vi "rechtdoor.vi"   [LabVIEW 2019]
uses:
  <vilib>/myRIO/Common/Instrument Driver Framework/Utilities/typedefs/Analog Scaling Constants.ctl
  <vilib>/myRIO/Common/Instrument Driver Framework/Utilities/typedefs/Analog Scaling Constants List.ctl
  <vilib>/myRIO/Common/Instrument Driver Framework/myRIO v1.0/AO/typedefs/AO Channels Enum.ctl
  <vilib>/myRIO/Common/Instrument Driver Framework/myRIO v1.0/AO/typedefs/AO Channels List.ctl
  <vilib>/myRIO/Common/Instrument Driver Framework/Utilities/typedefs/Generic FPGA Reference.ctl
  <vilib>/myRIO/Common/Instrument Driver Framework/Utilities/typedefs/myRIO v1.0 Reference.ctl
  <vilib>/myRIO/Common/Instrument Driver Framework/Utilities/typedefs/Hardware Version Enum.ctl
  <vilib>/myRIO/Common/Instrument Driver Framework/Utilities/typedefs/myRIO Generic Hardware Reference.ctl
  <vilib>/myRIO/Instrument Drivers/Onboard IO/AO/typedefs/AO Reference.ctl
  <vilib>/myRIO/Instrument Drivers/Onboard IO/AO/AO.lvlib
  <vilib>/myRIO/Instrument Drivers/Onboard IO/AO/vis/Write.vi
  <vilib>/userDefined/High Color/nirio_resource_hc.ctl
  <vilib>/myRIO/Common/Instrument Driver Framework/myRIO v1.0/AO/vis/myRIO v1.1 Open AO.vi
  <vilib>/myRIO/Instrument Drivers/Onboard IO/AO/vis/myRIO AO Open.xnode
  <vilib>/myRIO/Common/Instrument Driver Framework/Utilities/vis/Is FPGA Ref Available.vi
  <vilib>/myRIO/Express VI/Onboard IO/AO/AO Express VI.xnode
  <vilib>/myRIO/Common/Instrument Driver Framework/myRIO v1.0/DIO/typedefs/DIO Channels Enum.ctl
  <vilib>/myRIO/Common/Instrument Driver Framework/myRIO v1.0/DIO/typedefs/DIO Channels List.ctl
  <vilib>/myRIO/Instrument Drivers/Onboard IO/DIO/typedefs/DIO Reference.ctl
  <vilib>/myRIO/Instrument Drivers/Onboard IO/DIO/DIO.lvlib
  <vilib>/myRIO/Instrument Drivers/Onboard IO/DIO/vis/Read.vi
  <vilib>/myRIO/Instrument Drivers/Onboard IO/DIO/vis/myRIO DIO Open.xnode
  <vilib>/myRIO/Express VI/Onboard IO/DI/DI Express VI.xnode
  interface.vi
  <vilib>/myRIO/Common/Instrument Driver Framework/myRIO v1.0/DIO/vis/myRIO v1.1 Open DIO.vi
types:
  T1 = typedef "AO.lvlib/AO Reference.ctl" = cluster{"myRIO Reference":T2, "AO Channel List":T6, "AO Scaling Constant List":T8}
  T2 = typedef "myRIO Generic Hardware Reference.ctl" = cluster{"myRIO Model":T3, "myRIO Hardware Reference":T4}
  T3 = typedef "Hardware Version Enum.ctl" = enum16{"Unknown", "myRIO-1900", "myRIO-1950", "roboRIO", "NI ELVIS RIO CM", "ELVIS III"}
  T4 = typedef "myRIO v1.0 Reference.ctl" = cluster{"Generic FPGA Reference":T5, "Allow multiple opens":bool}
  T5 = typedef "Generic FPGA Reference.ctl" = refnum<k20>
  T6 = typedef "AO Channels List.ctl" = T7[]
  T7 = typedef "AO Channels Enum.ctl" = enum16{"Not Connected", "AudioOut/Left", "AudioOut/Right", "C/AO0", "C/AO1", "A/AO0", "A/AO1", "B/AO0", "B/AO1"}
  T8 = typedef "Analog Scaling Constants List.ctl" = T9[]
  T9 = typedef "Analog Scaling Constants.ctl" = cluster{"LSB Weight (Volts)":dbl, "Offset (Volts)":dbl, "Signed?":bool}
  T10 = typedef "nirio_resource_hc.ctl" = tag
  T11 = typedef "DIO.lvlib/DIO Reference.ctl" = cluster{"myRIO Reference":T2, "DIO Channels List":T12}
  T12 = typedef "DIO Channels List.ctl" = T13[]
  T13 = typedef "DIO Channels Enum.ctl" = enum16{"Not Connected", "C/DIO0", "C/DIO1", "C/DIO2", "C/DIO3", "C/DIO4", "C/DIO5", "C/DIO6", "C/DIO7", "A/DIO0", "A/DIO1", "A/DIO2", "A/DIO3", "A/DIO4", "A/DIO5", "A/DIO6", "A/DIO7", "A/DIO8", "A/DIO9", "A/DIO10", "A/DIO11", "A/DIO12", "A/DIO13", "A/DIO14", "A/DIO15", "A/DIO16", "A/DIO17", "A/DIO18", "A/DIO19", "B/DIO0", "B/DIO1", "B/DIO2", "B/DIO3", "B/DIO4", "B/DIO5", "B/DIO6", "B/DIO7", "B/DIO8", "B/DIO9", "B/DIO10", "B/DIO11", "B/DIO12", "B/DIO13", "B/DIO14", "B/DIO15", "B/DIO16", "B/DIO17", "B/DIO18", "B/DIO19", "LED0", "LED1", "LED2", "LED3", "Button0", "DIO/DIO0", "DIO/DIO1", "DIO/DIO2", "DIO/DIO3", "DIO/DIO4", "DIO/DIO5", "DIO/DIO6", "DIO/DIO7", "DIO/DIO8", "DIO/DIO9", "SPI/CS0", "SPI/CS1", "SPI/CS2", "SPI/CS3", "LED RADIO (Green)", "LED RADIO (Red)", "LED COMM (Green)", "LED COMM (Red)", "LED MODE (Green)", "LED MODE (Red)"}
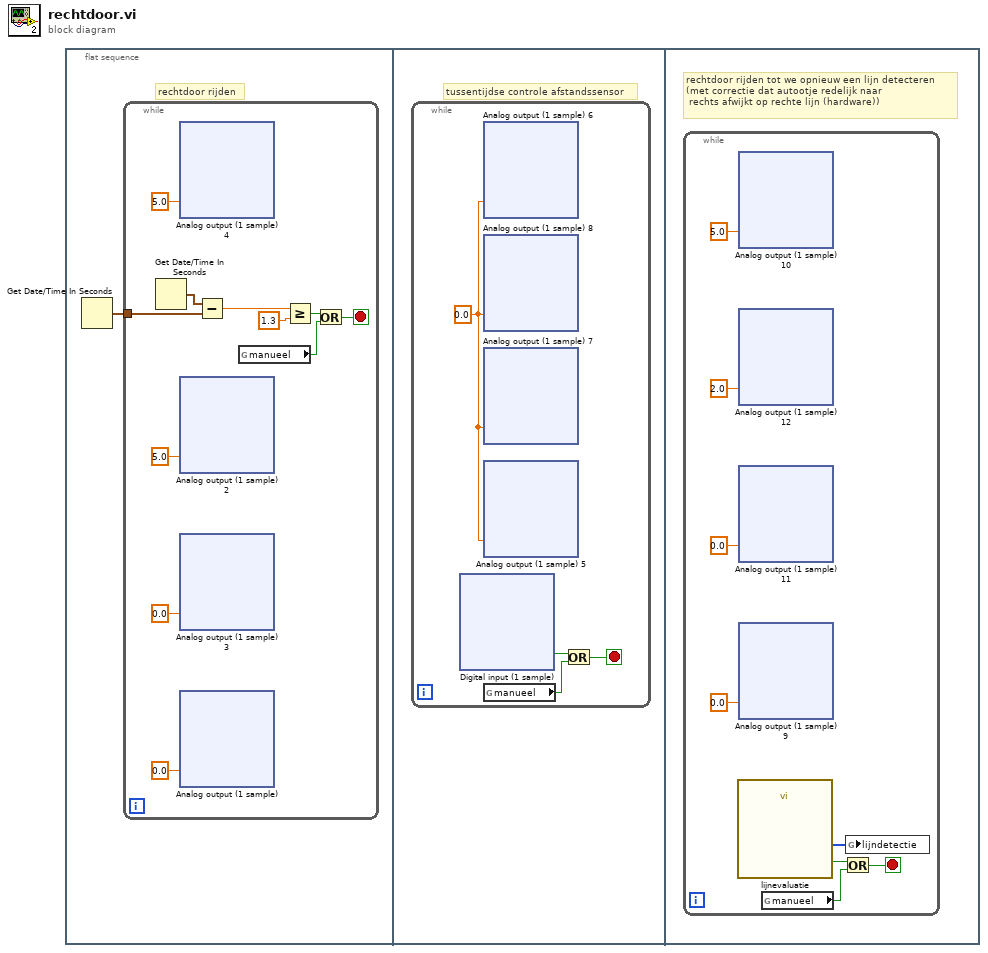
[diagram p0: block diagram]
diagram:
  n1 = flat-sequence {
    frame #0 {
      # "rechtdoor rijden"
      n2 = Get Date/Time In Seconds() -> (seconds since 1Jan1904=w1:timestamp)
      n3 = while {
        tunnel: w1 -> [w4]
        stop <- w7 stop-if-true
        n4 = Get Date/Time In Seconds() -> (seconds since 1Jan1904=w5:timestamp)
        n5 = xnode "Analog output (1 sample) 4"("A/AO0 (Pin 2)"=5.0) -> ()  [unwired: 1 in, 1 out]
        n6 = xnode "Analog output (1 sample) 2"("B/AO0 (Pin 2)"=5.0) -> ()  [unwired: 1 in, 1 out]
        n7 = xnode "Analog output (1 sample) 3"("A/AO1 (Pin 4)"=0.0) -> ()  [unwired: 1 in, 1 out]
        n8 = xnode "Analog output (1 sample)"("B/AO1 (Pin 4)"=0.0) -> ()  [unwired: 1 in, 1 out]
        n9 = Subtract(x=w5, y=w4) -> (x-y=w6:dbl)
        n10 = global read "interface.vi" "manueel"() -> (w8:bool)
        n11 = Greater Or Equal?(x=w6, y=1.3) -> (x >= y?=w3:bool)
        n12 = Or(x=w3, y=w8) -> (x .or. y?=w7:bool)
      }
    }
    frame #1 {
      # "tussentijdse controle afstandssensor"
      n13 = while {
        stop <- w162 stop-if-true
        w164 = 0.0
        n14 = xnode "Digital input (1 sample)"() -> ("A/DIO1 (Pin 13)"=w163:bool)  [unwired: 1 in, 1 out]
        n15 = xnode "Analog output (1 sample) 6"("A/AO1 (Pin 4)"=w164) -> ()  [unwired: 1 in, 1 out]
        n16 = xnode "Analog output (1 sample) 8"("B/AO0 (Pin 2)"=w164) -> ()  [unwired: 1 in, 1 out]
        n17 = xnode "Analog output (1 sample) 7"("A/AO0 (Pin 2)"=w164) -> ()  [unwired: 1 in, 1 out]
        n18 = xnode "Analog output (1 sample) 5"("B/AO1 (Pin 4)"=w164) -> ()  [unwired: 1 in, 1 out]
        n19 = global read "interface.vi" "manueel"() -> (w161:bool)
        n20 = Or(x=w163, y=w161) -> (x .or. y?=w162:bool)
      }
    }
    frame #2 {
      # "rechtdoor rijden tot we opnieuw een lijn detecteren\n(met correctie dat autootje redelijk naar\n rechts afwijkt op rechte lijn (hardware))"
      n21 = while {
        stop <- w353 stop-if-true
        n22 = call "lijnevaluatie.vi"() -> ("digitaal lijn 0-1"=w348:i32[], "lijn gedecteerd"=w349:bool)  [unwired: 8 in, 2 out]
        n23 = xnode "Analog output (1 sample) 10"("B/AO0 (Pin 2)"=5.0) -> ()  [unwired: 1 in, 1 out]
        n24 = xnode "Analog output (1 sample) 12"("A/AO0 (Pin 2)"=2.0) -> ()  [unwired: 1 in, 1 out]
        n25 = xnode "Analog output (1 sample) 11"("A/AO1 (Pin 4)"=0.0) -> ()  [unwired: 1 in, 1 out]
        n26 = xnode "Analog output (1 sample) 9"("B/AO1 (Pin 4)"=0.0) -> ()  [unwired: 1 in, 1 out]
        n27 = global read "interface.vi" "manueel"() -> (w352:bool)
        n28 = Or(x=w349, y=w352) -> (x .or. y?=w353:bool)
        n29 = global write "interface.vi" "lijndetectie"(w348) -> ()
      }
    }
  }
